vi "Release.vi"(8 "error in (no error)":errorcluster, 11 "TcpRouter-Client in":refnum<class "TcpRouter-Client.lvclass">) -> (0 "error out":errorcluster)   [LabVIEW 2020, in "CSM-TCP-Router.lvlib" / "TcpRouter-Client.lvclass"]
uses:
  TcpRouter-Client.lvclass
  TcpRouter-Client.lvclass/TcpRouter-Client.ctl
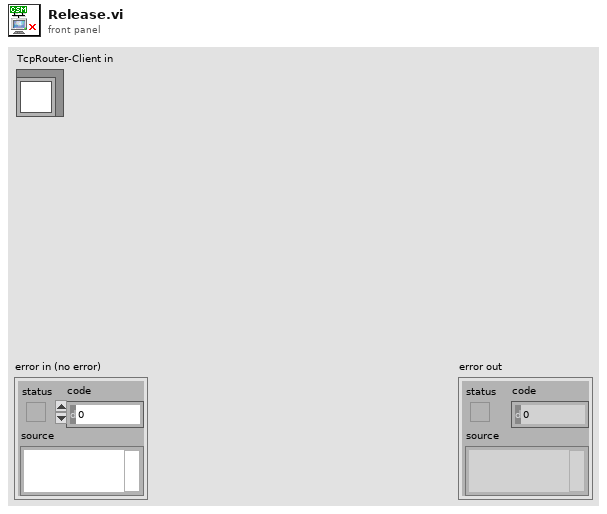
[diagram p1: front panel]
types:
  T1 = typedef "CSM-TCP-Router.lvlib/TcpRouter-Client.lvclass/Def-TCP-Router REQ-REP.ctl" = cluster{"REQ-REP":refnum<k5>}
  T2 = typedef "CSM-TCP-Router.lvlib/TcpRouter-Client.lvclass/Def-TCP-Router PUB-SUB.ctl" = cluster{"STATUS":refnum<k5>, "StatusQueue":refnum<queue>}
  T3 = typedef "CSM-TCP-Router.lvlib/TcpRouter-Client.lvclass/Def-TCP-Router ASYNC-RESP.ctl" = cluster{"Async-Resp":refnum<k5>, "RespQueue":refnum<queue>, "RespEvent":refnum<user-event>}
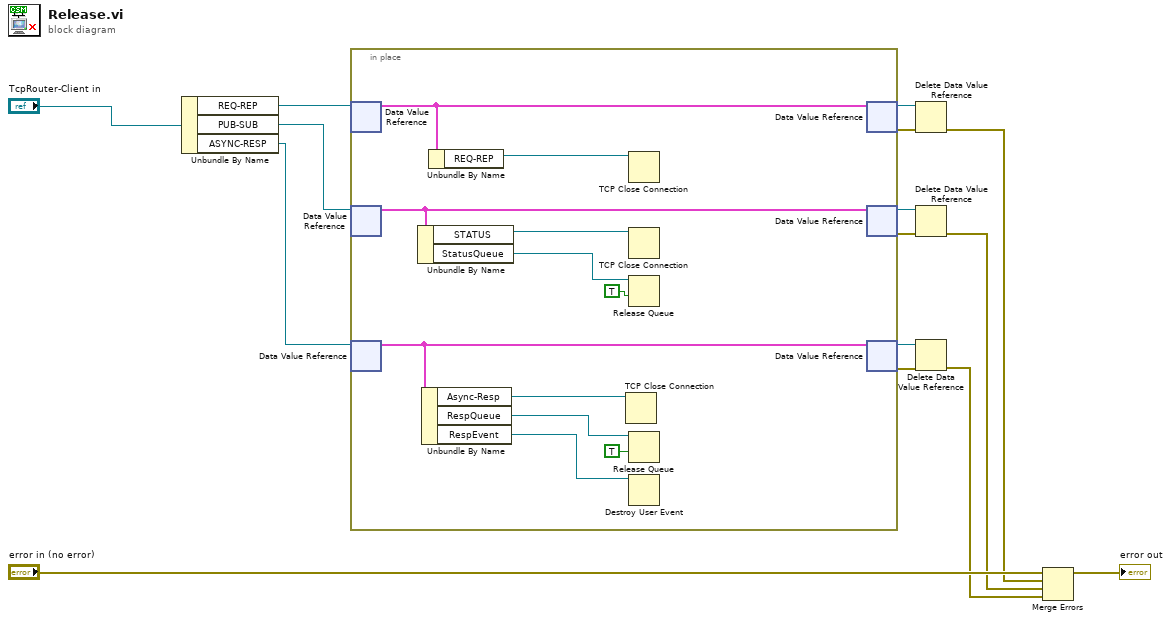
[diagram p0: block diagram]
diagram:
  n1 = Unbundle By Name("TcpRouter-Client in") -> ("REQ-REP"=w13:refnum<data-value>, "PUB-SUB"=w8:refnum<data-value>, "ASYNC-RESP"=w4:refnum<data-value>)
  n2 = in-place {
    n3 = in-place-dvr #1(w13) -> (w26:T1)  [unwired: 1 out]
    n4 = in-place-dvr #2(w8) -> (w23:T2)  [unwired: 1 out]
    n5 = in-place-dvr #3(w4) -> (w21:T3)  [unwired: 1 out]
    n6 = Unbundle By Name(w23) -> ("STATUS"=w24:refnum<k5>, "StatusQueue"=w22:refnum<queue>)
    n7 = Unbundle By Name(w21) -> ("Async-Resp"=w19:refnum<k5>, "RespQueue"=w20:refnum<queue>, "RespEvent"=w16:refnum<user-event>)
    n8 = Unbundle By Name(w26) -> ("REQ-REP"=w25:refnum<k5>)
    n9 = TCP Close Connection(connection ID=w19) -> ()  [unwired: 2 in, 2 out]
    n10 = TCP Close Connection(connection ID=w25) -> ()  [unwired: 2 in, 2 out]
    n11 = TCP Close Connection(connection ID=w24) -> ()  [unwired: 2 in, 2 out]
    n12 = Release Queue(queue=w22, force destroy? (F)=TRUE) -> ()  [unwired: 1 in, 3 out]
    n13 = Release Queue(queue=w20, force destroy? (F)=TRUE) -> ()  [unwired: 1 in, 3 out]
    n14 = Destroy User Event(user event=w16) -> ()  [unwired: 1 in, 1 out]
    n15 = in-place-dvr #1(w26) -> (w11:refnum<data-value>, w12:errorcluster)
    n16 = in-place-dvr #2(w23) -> (w6:refnum<data-value>, w7:errorcluster)
    n17 = in-place-dvr #3(w21) -> (w2:refnum<data-value>, w3:errorcluster)
  }
  n18 = Delete Data Value Reference(data value reference=w11, error in=w12) -> (error out=w9:errorcluster)  [unwired: 1 out]
  n19 = Delete Data Value Reference(data value reference=w6, error in=w7) -> (error out=w5:errorcluster)  [unwired: 1 out]
  n20 = Delete Data Value Reference(data value reference=w2, error in=w3) -> (error out=w1:errorcluster)  [unwired: 1 out]
  n21 = Merge Errors("error in (no error)", w9, w5, w1) -> (→"error out":errorcluster)
